vi "configure tdms channels.vi"(4 "samples per channel (1)":u32=1, 6 "type order":T1[](array[typedef]), 7 "group name":string, 8 "error in":errorcluster, 10 "dictionary":T2, 11 "tdms file in":refnum<k34>) -> (0 "error out":errorcluster, 3 "tdms file out":refnum<k34>)   [LabVIEW 2013, in "TDMS datalogger runtime.lvclass"]
uses:
  TDMS datalogger runtime.lvclass
  <vilib>/NI/Tag Bus/dictionary/full data dictionary.ctl
  <vilib>/NI/Tag Bus/tag/Data Type.ctl
  <vilib>/NI/Tag Bus/tag/tag descriptor.lvclass
  <vilib>/NI/Tag Bus/dictionary/data dictionary.lvclass
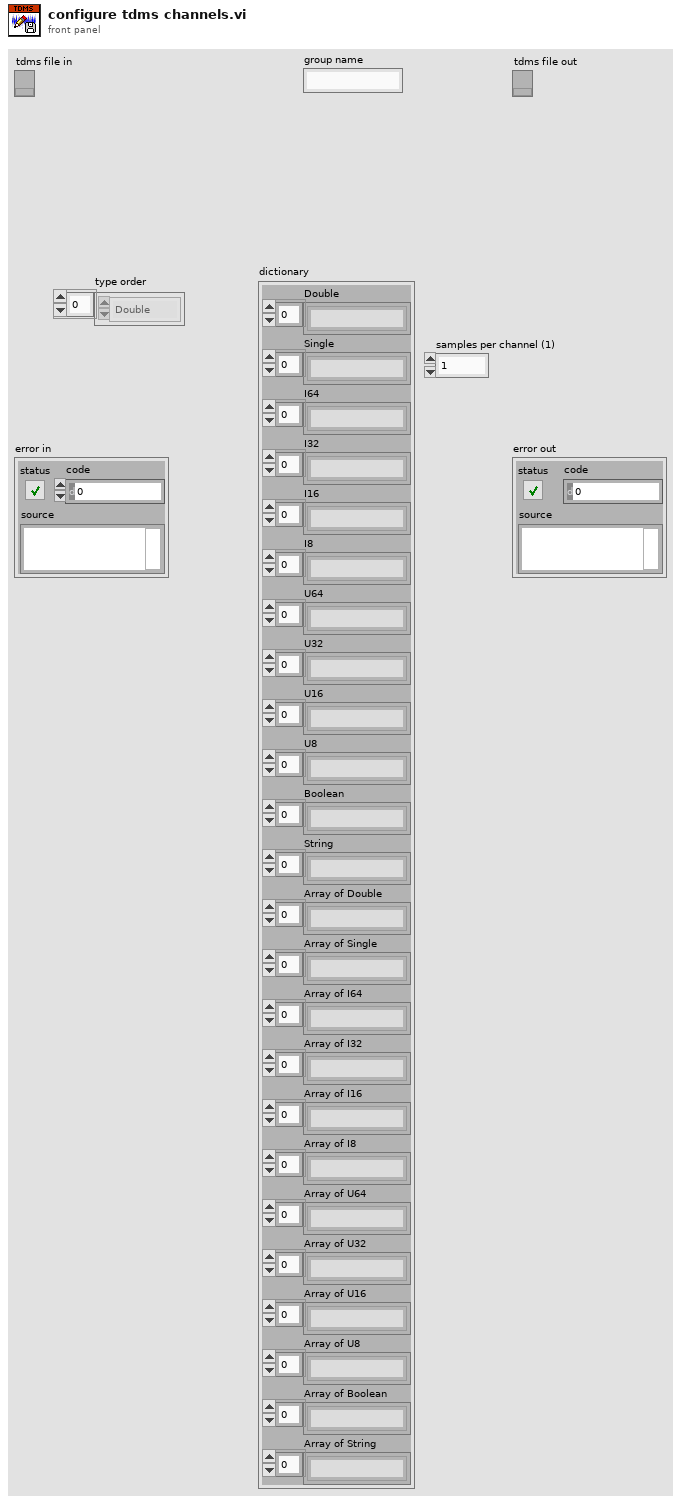
[diagram p1: front panel]
types:
  T1 = typedef "tag bus.lvlib/tag descriptor.lvclass/Data Type.ctl" = enum16{"Double", "Single", "I64", "I32", "I16", "I8", "U64", "U32", "U16", "U8", "Boolean", "String", "Array of Double", "Array of Single", "Array of I64", "Array of I32", "Array of I16", "Array of I8", "Array of U64", "Array of U32", "Array of U16", "Array of U8", "Array of Boolean", "Array of String"}
  T2 = typedef "tag bus.lvlib/data dictionary.lvclass/full data dictionary.ctl" = cluster{"Double":string[], "Single":string[], "I64":string[], "I32":string[], "I16":string[], "I8":string[], "U64":string[], "U32":string[], "U16":string[], "U8":string[], "Boolean":string[], "String":string[], "Array of Double":string[], "Array of Single":string[], "Array of I64":string[], "Array of I32":string[], "Array of I16":string[], "Array of I8":string[], "Array of U64":string[], "Array of U32":string[], "Array of U16":string[], "Array of U8":string[], "Array of Boolean":string[], "Array of String":string[]}
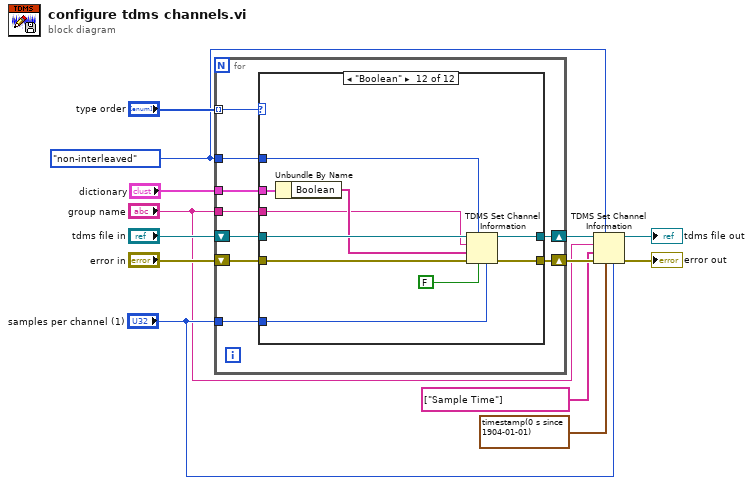
[diagram p0: block diagram]
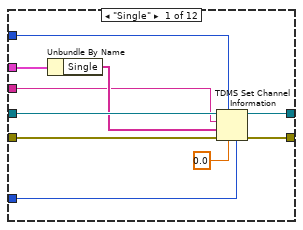
[diagram p2: hidden frame]
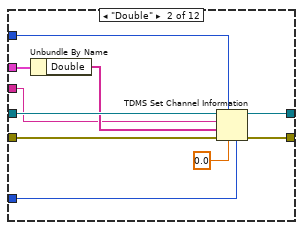
[diagram p3: hidden frame]
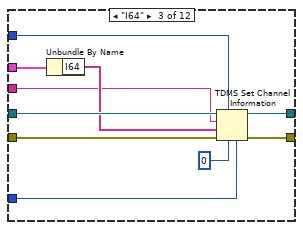
[diagram p4: hidden frame]
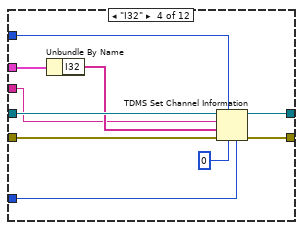
[diagram p5: hidden frame]
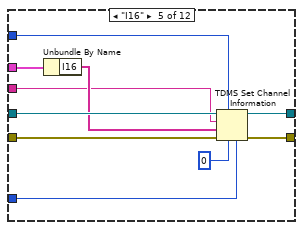
[diagram p6: hidden frame]
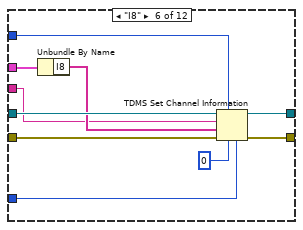
[diagram p7: hidden frame]
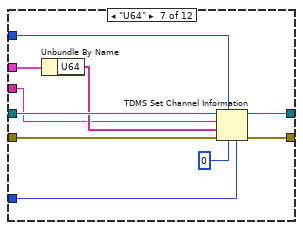
[diagram p8: hidden frame]
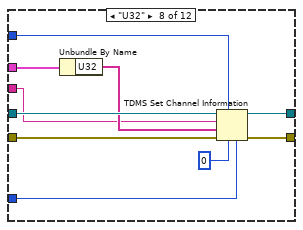
[diagram p9: hidden frame]
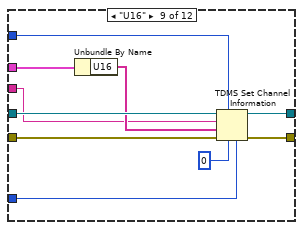
[diagram p10: hidden frame]
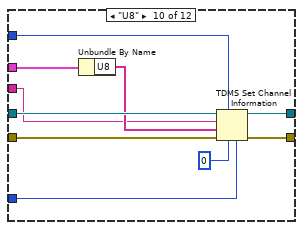
[diagram p11: hidden frame]
diagram:
  w5 = enum16{"non-interleaved", "interleaved"}."non-interleaved" ("data layout (0:non-interleaved)")
  n1 = for {
    tunnel: "dictionary" -> [w15]
    shift-right: [w21] -> w12
    shift-left: "error in" -> [w22]
    shift-right: [w19] -> w7
    shift-left: "tdms file in" -> [w20]
    tunnel: w5 -> [w18]
    tunnel: "samples per channel (1)" -> [w17]
    tunnel: "type order" -> [w16] mode=indexing
    tunnel: "group name" -> [w14]
    n2 = case shown="\"Boolean\"" w16 {
      tunnel: w22 -> [w32 w42 w52 w62 w72 w82 w92 w102 w112 w122 w124 w134]
      tunnel: [w31 w41 w51 w61 w71 w81 w91 w101 w111 w121 w124 w133] -> w21
      tunnel: w20 -> [w30 w40 w50 w60 w70 w80 w90 w100 w110 w120 w123 w132]
      tunnel: [w29 w39 w49 w59 w69 w79 w89 w99 w109 w119 w123 w131] -> w19
      tunnel: w18 -> [w27 w37 w47 w57 w67 w77 w87 w97 w107 w117 _ w129]
      tunnel: w17 -> [w26 w36 w46 w56 w66 w76 w86 w96 w106 w116 _ w128]
      tunnel: w15 -> [w25 w35 w45 w55 w65 w75 w85 w95 w105 w115 _ w127]
      tunnel: w14 -> [w23 w33 w43 w53 w63 w73 w83 w93 w103 w113 _ w125]
      frame "Single" {
        n3 = Unbundle By Name(w25) -> ("Single"=w24:string[])
        n4 = TDMS Set Channel Information(4:w26, 6:sgl 0.0, 7:w27, 8:w32, 9:w24, 10:w23, 11:w30) -> (0:w31:errorcluster, 3:w29:refnum<k34>)
      }
      frame "Double" {
        n5 = Unbundle By Name(w35) -> ("Double"=w34:string[])
        n6 = TDMS Set Channel Information(4:w36, 6:0.0, 7:w37, 8:w42, 9:w34, 10:w33, 11:w40) -> (0:w41:errorcluster, 3:w39:refnum<k34>)
      }
      frame "I64" {
        n7 = Unbundle By Name(w45) -> ("I64"=w44:string[])
        n8 = TDMS Set Channel Information(4:w46, 6:i64 0, 7:w47, 8:w52, 9:w44, 10:w43, 11:w50) -> (0:w51:errorcluster, 3:w49:refnum<k34>)
      }
      frame "I32" {
        n9 = Unbundle By Name(w55) -> ("I32"=w54:string[])
        n10 = TDMS Set Channel Information(4:w56, 6:0, 7:w57, 8:w62, 9:w54, 10:w53, 11:w60) -> (0:w61:errorcluster, 3:w59:refnum<k34>)
      }
      frame "I16" {
        n11 = Unbundle By Name(w65) -> ("I16"=w64:string[])
        n12 = TDMS Set Channel Information(4:w66, 6:i16 0, 7:w67, 8:w72, 9:w64, 10:w63, 11:w70) -> (0:w71:errorcluster, 3:w69:refnum<k34>)
      }
      frame "I8" {
        n13 = Unbundle By Name(w75) -> ("I8"=w74:string[])
        n14 = TDMS Set Channel Information(4:w76, 6:i8 0, 7:w77, 8:w82, 9:w74, 10:w73, 11:w80) -> (0:w81:errorcluster, 3:w79:refnum<k34>)
      }
      frame "U64" {
        n15 = Unbundle By Name(w85) -> ("U64"=w84:string[])
        n16 = TDMS Set Channel Information(4:w86, 6:u64 0, 7:w87, 8:w92, 9:w84, 10:w83, 11:w90) -> (0:w91:errorcluster, 3:w89:refnum<k34>)
      }
      frame "U32" {
        n17 = Unbundle By Name(w95) -> ("U32"=w94:string[])
        n18 = TDMS Set Channel Information(4:w96, 6:u32 0, 7:w97, 8:w102, 9:w94, 10:w93, 11:w100) -> (0:w101:errorcluster, 3:w99:refnum<k34>)
      }
      frame "U16" {
        n19 = Unbundle By Name(w105) -> ("U16"=w104:string[])
        n20 = TDMS Set Channel Information(4:w106, 6:u16 0, 7:w107, 8:w112, 9:w104, 10:w103, 11:w110) -> (0:w111:errorcluster, 3:w109:refnum<k34>)
      }
      frame "U8" {
        n21 = Unbundle By Name(w115) -> ("U8"=w114:string[])
        n22 = TDMS Set Channel Information(4:w116, 6:u8 0, 7:w117, 8:w122, 9:w114, 10:w113, 11:w120) -> (0:w121:errorcluster, 3:w119:refnum<k34>)
      }
      frame Default {
      }
      frame "Boolean" {
        n23 = Unbundle By Name(w127) -> ("Boolean"=w126:string[])
        n24 = TDMS Set Channel Information(4:w128, 6:FALSE, 7:w129, 8:w134, 9:w126, 10:w125, 11:w132) -> (0:w133:errorcluster, 3:w131:refnum<k34>)
      }
    }
  }
  n25 = TDMS Set Channel Information(4:"samples per channel (1)", 6:timestamp(0 s since 1904-01-01), 7:w5, 8:w12, 9:string[] ["Sample Time"] ("channel name(s)"), 10:"group name", 11:w7) -> (0:→"error out":errorcluster, 3:→"tdms file out":refnum<k34>)
